vi "Read from LPC.vi"(8 "error in (no error)":errorcluster, 11 "VISA resource name":refnum<visa-resource-name>="GPIB0::3::INSTR") -> (0 "error out":errorcluster, 1 "control mode":T1(ring), 2 "wavelength":dbl[unit], 3 "VISA resource name out":refnum<visa-resource-name>, 4 "front-panel controls":enum16{"enabled", "disabled"}(ring), 5 "power":dbl[unit])   [LabVIEW 2009, in "BEOC LPC.lvlib"]
doc: "Reads the most important settings from the LPC (laser power controller)."
uses:
  BEOC LPC.lvlib
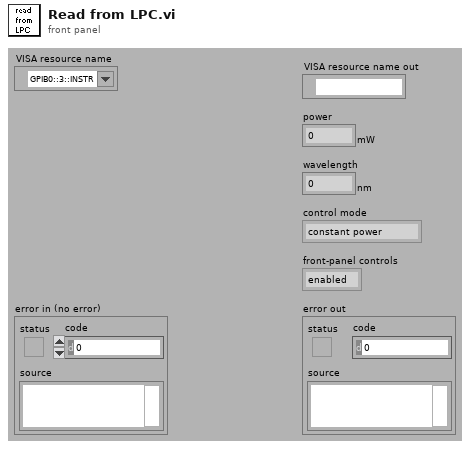
[diagram p1: front panel]
types:
  T1 = enum16{"constant power", "constant transmission"}
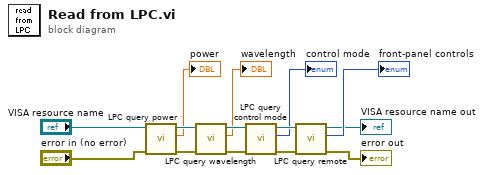
[diagram p0: block diagram]
diagram:
  n1 = call "LPC query power.vi"("error in (no error)"="error in (no error)", "VISA resource name"="VISA resource name") -> ("error out"=w12:errorcluster, "power"=→"power":dbl[unit], "VISA resource name out"=w9:refnum<visa-resource-name>)  [unwired: 7 out]
  n2 = call "LPC query wavelength.vi"("error in (no error)"=w12, "VISA resource name"=w9) -> ("error out"=w11:errorcluster, "wavelength"=→"wavelength":dbl[unit], "VISA resource name out"=w8:refnum<visa-resource-name>)  [unwired: 7 out]
  n3 = call "LPC query control mode.vi"("error in (no error)"=w11, "VISA resource name"=w8) -> ("error out"=w10:errorcluster, "control mode"=→"control mode":T1, "VISA resource name out"=w7:refnum<visa-resource-name>)  [unwired: 7 out]
  n4 = call "LPC query remote.vi"("error in (no error)"=w10, "VISA resource name"=w7) -> ("error out"=→"error out":errorcluster, "front-panel controls"=→"front-panel controls":enum16{"enabled", "disabled"}, "VISA resource name out"=→"VISA resource name out":refnum<visa-resource-name>)  [unwired: 7 out]
